vi "Read from Text File.vi"(8 "error in":errorcluster, 11 "file path (use dialog)":path=path "C:/CoMP-S Observer/focus.txt") -> (0 "error out":errorcluster, 2 "Data String":string, 3 "number":ext)   [LabVIEW 2014]
doc: "Reads a text file created by the Write to Text File VI in this LLB and plots the data. The VI reads one line at a time, splits off the first (timestamp) column from the subsequent data columns, and converts the data to numbers and plots them. Refer to the sprdsht.llb for an example of the spreadsheet format."
panel:
  # "Return read value from text file and transform to EXT type of Number"
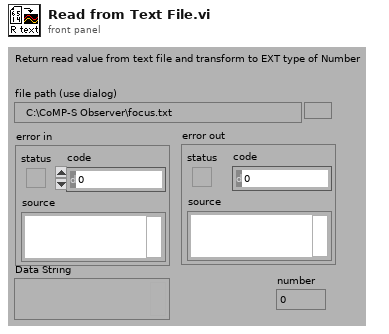
[diagram p1: front panel]
types:
  T1 = enum16{"open", "replace", "create", "open or create", "replace or create", "replace or create with confirmation"}
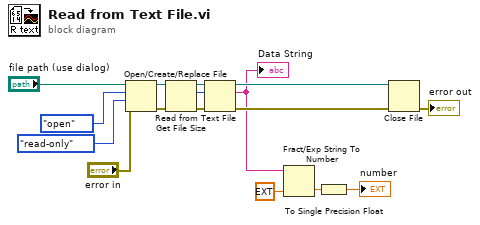
[diagram p0: block diagram]
diagram:
  n1 = Open/Create/Replace File(file path (use dialog)="file path (use dialog)", error in="error in", operation (0:open)=T1."open", access (0:read/write)=enum16{"read/write", "read-only", "write-only"}."read-only") -> (refnum out=w12:refnum<file>, error out=w13:errorcluster)  [unwired: 3 out]
  n2 = Get File Size(file=w12, error in=w13) -> (refnum out=w11:refnum<file>, size (in bytes)=w10:i64, 0:w9:errorcluster)
  n3 = Read from Text File(file (use dialog)=w11, count=w10, error in=w9) -> (refnum out=w16:refnum<file>, text=w5:string, error out=w15:errorcluster)  [unwired: 2 out]
  "Data String" <- w5
  n4 = Fract/Exp String To Number(string=w5, default (0 dbl)=ext 0.0 ("default (0 DBL)")) -> (number=w1:ext)  [unwired: 2 in, 1 out]
  n5 = To Single Precision Float(number=w1) -> (single precision float=→"number":sgl)
  n6 = Close File(refnum=w16, error in=w15) -> (error out=→"error out":errorcluster)  [unwired: 1 out]
